vi "that_amazing.vi"() -> ()   [LabVIEW 2024]
panel:
  in  "Setup":T1={"Scaling (pixels/mm)"=1.0, "Tool Diameter (inch)"=0.25, "Origin location"={"x (mm)"=10, "y (mm)"=315}, "Wood dim"={"width (inch)"=10.0, "height (inch)"=12.0}}
  out "Mouse coordinates":cluster{"X (mm)":dbl, "Y (mm)":dbl}
  out "Position 3":T2
  in  "Manual Input":cluster{"x":dbl, "y":dbl}[](array[cluster])
  in  "Timeout (ms)":u32=1000
  in  "VISA Refnum in 2":refnum<visa-resource-name>="COM9"
  in  "Realtime control":bool
  in  "Manual or Gcode":bool=TRUE
  in  "Velocity control":bool
  in  "L 2":dbl(slide)=80.0 scale=0.0..200.0
  in  "L 1":dbl(slide)=80.0 scale=0.0..200.0
  in  "file (use dialog)":path=path "D:/Tufts/ME121/Gcode/bird - Copy.gcode"
  out "end effector":cluster{dbl, dbl}={159.01647214211073, 1.9100783062530127} {"?" format="%.1f"; "?" format="%#.1f"}
  out "2D Kai Smith":picture
  in  "2D Pict origin":cluster{"x":dbl, "y":dbl}={"x"=200.0, "y"=200.0}
  # "2D-Arm Simulation & Control"
  # "mm"
  # "mm"
  # "mm"
  # "mm"
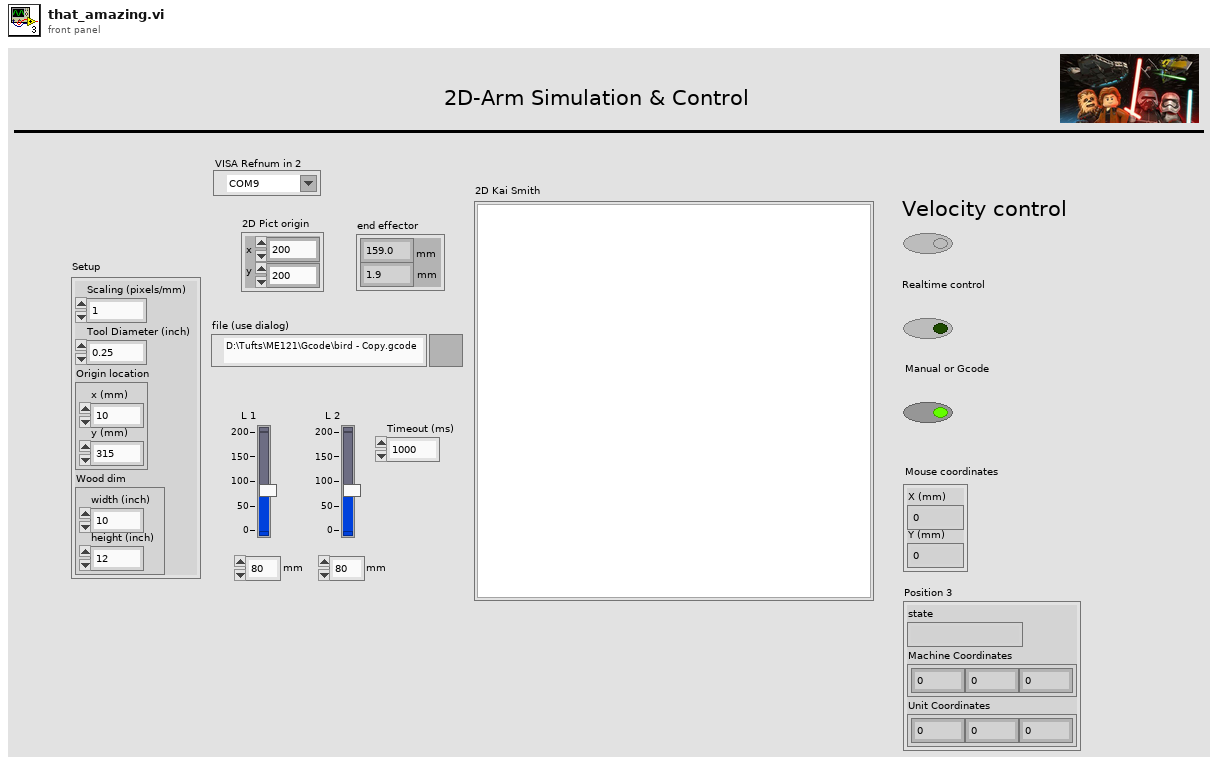
[diagram p1: front panel]
types:
  T1 = cluster{"Scaling (pixels/mm)":dbl, "Tool Diameter (inch)":dbl, "Origin location":cluster{"x (mm)":i16, "y (mm)":i16}, "Wood dim":cluster{"width (inch)":dbl, "height (inch)":dbl}}
  T2 = cluster{"state":string, "Machine Coordinates":cluster{"X":dbl, "Y":dbl, "Z":dbl}, "Unit Coordinates":cluster{"X":dbl, "Y":dbl, "Z":dbl}}
  T3 = typedef "LVPositionTypeDef.ctl" = cluster{"Left":i32, "Top":i32}
  T4 = typedef "LVMouseTypeDef.ctl" = cluster{"Mouse Position":cluster{"X":i32, "Y":i32}, "Mouse Modifiers":cluster{"Button Down":bool, "Shift Mod":bool, "Menu Mod":bool, "Option Mod":bool}}
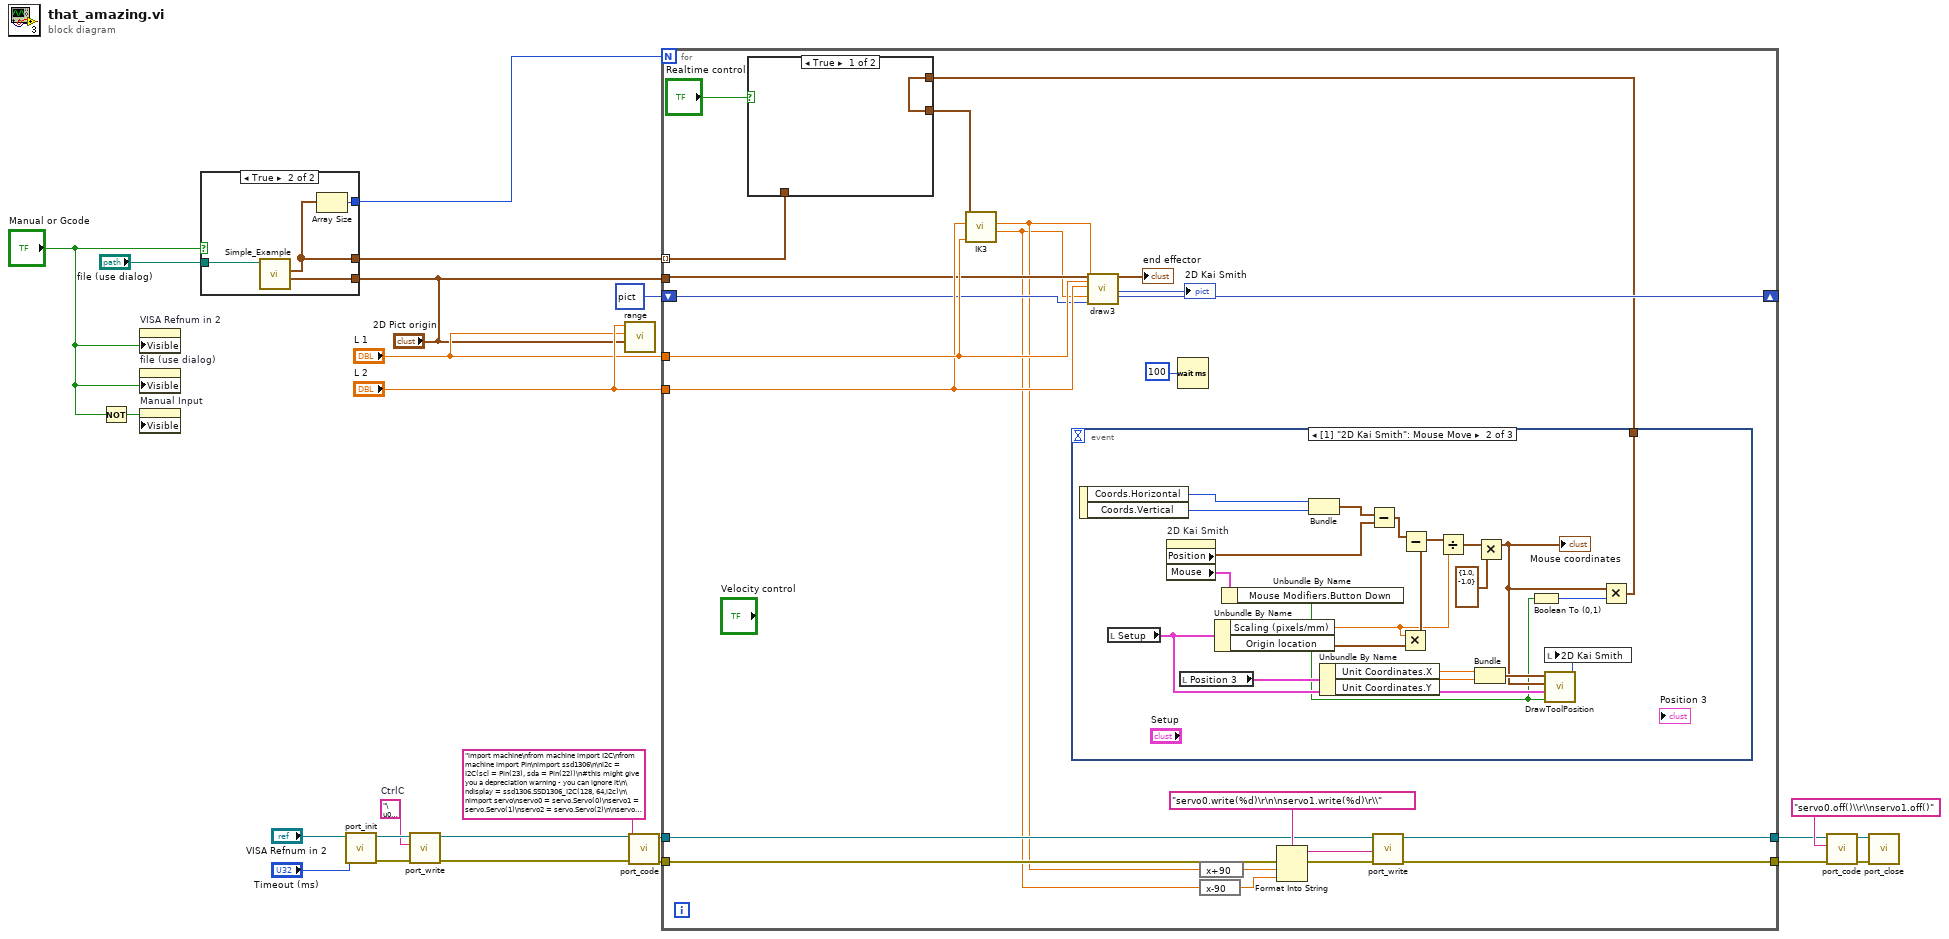
[diagram p0: block diagram]
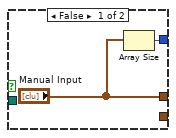
[diagram p2: hidden frame]
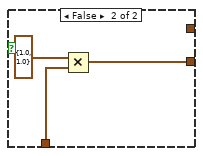
[diagram p3: hidden frame]
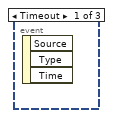
[diagram p4: hidden frame]
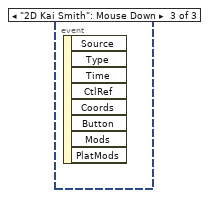
[diagram p5: hidden frame]
diagram:
  w14 = "\u0003"  # CtrlC
  n1 = Not(x="Manual or Gcode") -> (.not. x?=w4:bool)
  n2 = property on="VISA Refnum in 2" class="VISAName"("Visible"="Manual or Gcode") -> ()  [unwired: 2 in, 2 out]
  n3 = property on="file (use dialog)" class="Path"("Visible"="Manual or Gcode") -> ()  [unwired: 2 in, 2 out]
  n4 = property on="Manual Input" class="Arr (strict)"("Visible"=w4) -> ()  [unwired: 2 in, 2 out]
  n5 = case shown="True" "Manual or Gcode" {
    tunnel: "2D Pict origin" -> [_ w30]
    tunnel: ["Manual Input" w28] -> w20
    tunnel: [w26 w29] -> w5
    tunnel: "file (use dialog)" -> [_ w27]
    frame False {
      n6 = Array Size(array="Manual Input") -> (size(s)=w26:i32)
    }
    frame True {
      n7 = call <userlib>:"Simple_Example.vi"("2D Pict origin"=w30, "file (use dialog)"=w27) -> ("xy coord"=w28:cluster{"x":dbl, "y":dbl}[])  [unwired: 8 in, 1 out]
      n8 = Array Size(array=w28) -> (size(s)=w29:i32)
    }
  }
  n9 = call <userlib>:"port_init.vi"("Timeout (ms)"="Timeout (ms)", "VISA Refnum in"="VISA Refnum in 2") -> ("error out"=w17:errorcluster, "VISA Refnum out"=w18:refnum<visa-resource-name>)  [unwired: 8 in]
  n10 = call <userlib>:"port_write.vi"("error in (no error)"=w17, "write buffer"=w14, "VISA Refnum in"=w18) -> ("error out"=w15:errorcluster, "VISA Refnum out"=w16:refnum<visa-resource-name>)  [unwired: 7 in]
  n11 = call "range.vi"("2D Pict origin"="2D Pict origin", "L 1"="L 1", "L 2"="L 2") -> ()  [unwired: 8 in, 1 out]
  n12 = call <userlib>:"port_code.vi"("error in (no error)"=w15, "Code to run"="import machine\nfrom machine import I2C\nfrom machine import Pin\nimport ssd1306\n\ni2c = I2C(scl = Pin(23), sda = Pin(22))\n#this might give you a depreciation warning - you can ignore it\n\ndisplay = ssd1306.SSD1306_I2C(128, 64,i2c)\n\nimport servo\nservo0 = servo.Servo(0)\nservo1 = servo.Servo(1)\nservo2 = servo.Servo(2)\n\nservo0.write(90)\nservo1.write(90)\nservo2.write(90)\n\ndisplay.rect(10,10,60,50,1)\ndisplay.text('Good Aorning', 0, 0, 1)\ndisplay.show()\n    ", "VISA Refnum in"=w16) -> ("error out"=w6:errorcluster, "VISA Refnum out"=w7:refnum<visa-resource-name>)  [unwired: 7 in]
  n13 = for {
    N: w5 -> [_]
    tunnel: "2D Pict origin" -> [w46]
    shift-right: [w47] -> _
    shift-left: picture data[5B] ("new picture") -> [w49]
    tunnel: "L 1" -> [w51]
    tunnel: "L 2" -> [w50]
    tunnel: w20 -> [w33] mode=indexing
    tunnel: [w40] -> w9
    tunnel: [w39] -> w8
    tunnel: w7 -> [w38]
    tunnel: w6 -> [w37]
    n14 = event shown="[1] \"2D Kai Smith\": Mouse Move" {
      selector: _ -> [_ _ _]
      dyn-events: _ -> [_ _ _]
      timeout: _ -> [_ _ _]
      tunnel: [_ w58 _] -> w31
      event Timeout {
        n15 = event-data() -> ()  [unwired: 1 in, 3 out]
      }
      event "2D Kai Smith": Mouse Move {
        n16 = event-data() -> ("Coords.Horizontal"=w66:i32, "Coords.Vertical"=w65:i32)  [unwired: 1 in]
        n17 = local read "Setup"() -> (w62:T1)
        n18 = property on="2D Kai Smith" class="Pict"() -> ("Position"=w64:T3, "Mouse"=w63:T4)  [unwired: 2 in, 2 out]
        n19 = local read "Position 3"() -> (w72:T2)
        n20 = Unbundle By Name(w62) -> ("Scaling (pixels/mm)"=w75:dbl, "Origin location"=w78:cluster{"x (mm)":i16, "y (mm)":i16})
        n21 = Unbundle By Name(w63) -> ("Mouse Modifiers.Button Down"=w60:bool)
        n22 = Bundle("Horizontal"=w66, "Vertical"=w65) -> (w67:cluster{"Horizontal":i32, "Vertical":i32})  [unwired: 1 in]
        n23 = Unbundle By Name(w72) -> ("Unit Coordinates.X"=w70:dbl, "Unit Coordinates.Y"=w69:dbl)
        n24 = Subtract(x=w67, y=w64) -> (x-y=w74:T3)
        n25 = Multiply(x=w75, y=w78) -> (x*y=w77:cluster{"x (mm)":dbl, "y (mm)":dbl})
        n26 = Subtract(x=w74, y=w77) -> (x-y=w76:cluster{dbl, dbl})
        n27 = Divide(x=w76, y=w75) -> (x/y=w79:cluster{dbl, dbl})
        n28 = Bundle("X"=w70, "Y"=w69) -> (w68:cluster{"X":dbl, "Y":dbl})  [unwired: 1 in]
        n29 = Multiply(x=w79, y=cluster{dbl, dbl} {1.0, -1.0}) -> (x*y=w61:cluster{dbl, dbl})
        "Mouse coordinates" <- w61
        n30 = Boolean To (0,1)(Boolean=w60) -> (0, 1=w59:i16)
        n31 = call "DrawToolPosition.vi"("Show lines"=w60, "Setup"=w62, "mouse position"=w61, "dot position"=w68) -> ("blob"=w71:picture)  [unwired: 7 in]
        n32 = local write "2D Kai Smith"(w71) -> ()
        n33 = Multiply(x=w61, y=w59) -> (x*y=w58:cluster{dbl, dbl})
      }
      event "2D Kai Smith": Mouse Down {
        n34 = event-data() -> ()  [unwired: 1 in, 8 out]
      }
    }
    n35 = case shown="True" "Realtime control" {
      tunnel: w33 -> [_ w57]
      tunnel: [w54 w55] -> w32
      tunnel: w31 -> [w54 _]
      frame True {
      }
      frame False {
        n36 = Multiply(x=cluster{dbl, dbl} {1.0, 1.0}, y=w57) -> (x*y=w55:cluster{dbl, dbl})
      }
    }
    n37 = call "IK3.vi"("L1"=w51, "L2"=w50, "coordinates"=w32) -> ("theta21"=w35:dbl, "theta11"=w36:dbl)  [unwired: 6 in, 1 out]
    n38 = call "draw3.vi"("new position"=w46, "L 1"=w51, "L 2"=w50, "Angle1"=w36, "Angle 2"=w35, "input pic in loop"=w49) -> ("end effector"=→"end effector":cluster{dbl, dbl}, "2D Picture"=→"2D Kai Smith":picture, "shift pic"=w47:picture)  [unwired: 9 in, 2 out]
    n39 = Wait (ms)(milliseconds to wait=u32 100) -> ()  [unwired: 1 out]
    n40 = expression code="x+90"(w36) -> (w44:dbl)
    n41 = expression code="x-90"(w35) -> (w45:dbl)
    n42 = Format Into String(format string="servo0.write(%d)\r\n\nservo1.write(%d)\r\\", error in=w37, w44, w45) -> (resulting string=w43:string, error out=w42:errorcluster)  [unwired: 1 in]
    n43 = call <userlib>:"port_write.vi"("error in (no error)"=w42, "write buffer"=w43, "VISA Refnum in"=w38) -> ("error out"=w39:errorcluster, "VISA Refnum out"=w40:refnum<visa-resource-name>)  [unwired: 7 in]
  }
  n44 = call <userlib>:"port_code.vi"("error in (no error)"=w8, "Code to run"="servo0.off()\\r\\nservo1.off()", "VISA Refnum in"=w9) -> ("error out"=w10:errorcluster, "VISA Refnum out"=w11:refnum<visa-resource-name>)  [unwired: 7 in]
  n45 = call <userlib>:"port_close.vi"("error in (no error)"=w10, "VISA Refnum in"=w11) -> ()  [unwired: 10 in]
